vi "Digital Read.vi"(8 "Error In":errorcluster, 10 "DIO Channels":u8[](array[numeric]), 11 "LINX Device Config":T1) -> (0 "Error Out":errorcluster, 2 "Values":bool[](array[boolean]), 3 "LINX Device Config":T1)   [LabVIEW 2020, in "LMH-LINX.lvlib" / "Device.lvlib"]
uses:
  Device.lvlib
  Type Defs/LINX Device Config.ctl
  Type Defs/Interface.ctl
  Type Defs/TCP Config.ctl
  Type Defs/Channels.ctl
  Type Defs/Error Type.ctl
  LMH-LINX.lvlib
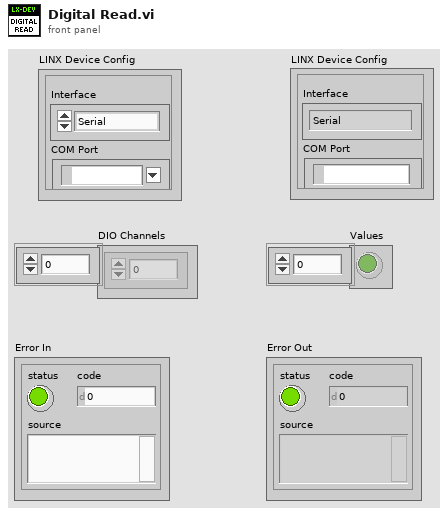
[diagram p1: front panel]
types:
  T1 = typedef "LMH-LINX.lvlib/Device.lvlib/LINX Device Config.ctl" = cluster{"Interface":T2, "COM Port":refnum<visa-resource-name>, "TCP Configuration":T3, "Device Family":u8, "Device ID":u8, "Device Name":string, "TCP Ref":refnum<k5>, "Channels":T4}
  T2 = typedef "LMH-LINX.lvlib/Interface.ctl" = enum16{"Serial", "TCP"}
  T3 = typedef "LMH-LINX.lvlib/Device.lvlib/TCP Config.ctl" = cluster{"IP Address":string, "Port":u16}
  T4 = typedef "LMH-LINX.lvlib/Channels.ctl" = cluster{"DI":u8[], "DO":u8[], "AI":u8[], "AO":u8[], "PWM":u8[], "QE":u8[], "UART":u8[], "I2C 2":u8[], "SPI":u8[], "CAN":u8[], "Servo":u8[], "AI Ref (V)":dbl, "AI Resolution (Bits)":u8, "AO Ref (V)":dbl, "AO Resolution (Bits)":u8}
  T5 = typedef "LMH-LINX.lvlib/Error Type.ctl" = enum16{"Unknown", "Timeout", "Corrupt Return Packet", "Unable To Connect", "Command Not Supported", "Channel DNE", "Invalid COM Config", "Firmware Version Mismatch", "myRIO Support", "CMD Specific Error", "Local IO Not Supported"}
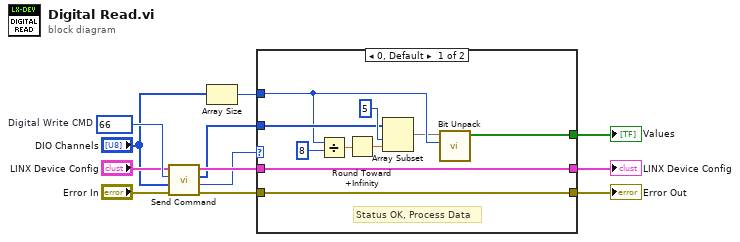
[diagram p0: block diagram]
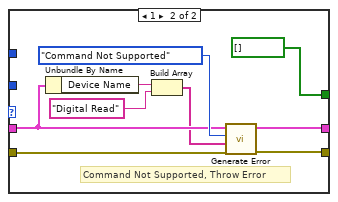
[diagram p2: hidden frame]
diagram:
  w11 = u16 66  # Digital Write CMD
  n1 = call "Send Command.vi"("Error In"="Error In", "ARGS"="DIO Channels", "CMD"=w11, "LINX Device Config"="LINX Device Config") -> ("Error Out"=w6:errorcluster, "Status"=w1:u8, "Response"=w5:u8[], "LINX Device Config"=w8:T1)  [unwired: 4 in]
  n2 = Array Size(array="DIO Channels") -> (size(s)=w3:i32)
  n3 = case shown="0, Default" w1 {
    tunnel: [w22 w29] -> w9
    tunnel: w8 -> [w22 w24]
    tunnel: [w21 w30] -> w7
    tunnel: w6 -> [w21 w31]
    tunnel: w5 -> [w15 _]
    tunnel: w3 -> [w14 _]
    tunnel: [w20 bool[] []] -> w2
    frame 0, Default {
      # "Status OK, Process Data"
      n4 = Divide(x=w14, y=8) -> (x/y=w17:dbl)
      n5 = Round Toward +Infinity(x=w17) -> (ceil(x): smallest int >= x=w18:dbl)
      n6 = Array Subset(array=w15, index=5, length=w18) -> (w13:u8[])
      n7 = call "Bit Unpack.vi"("Num Bits"=w14, "Data"=w13) -> ("Unpacked Data"=w20:bool[])  [unwired: 9 in]
    }
    frame 1 {
      # "Command Not Supported, Throw Error"
      n8 = Unbundle By Name(w24) -> ("Device Name"=w26:string)
      n9 = Build Array(w26, "Digital Read") -> (w23:string[])
      n10 = call "Generate Error.vi"("Error In"=w31, "Arguments"=w23, "Error Type"=Error_Type."Command Not Supported", "LINX Device Config"=w24) -> ("Error Out"=w30:errorcluster, "Dup LINX Device Config"=w29:T1)  [unwired: 6 in]
    }
  }
  "Error Out" <- w7
  "LINX Device Config" <- w9
  "Values" <- w2
